vi "getColumn.vi"(0 "reference in":refnum<class "python.lvclass">, 1 "filePath":string, 2 "sheetName":string, 3 "column":string, 4 "row":string, 5 "error in (no error)":errorcluster) -> (14 "reference out":refnum<class "python.lvclass">, 16 "data":string[](array[string]), 19 "error out":errorcluster)   [LabVIEW 2015, in "python.lvclass"]
uses:
  python.lvclass
  <vilib>/Utility/error.llb/DialogType.ctl
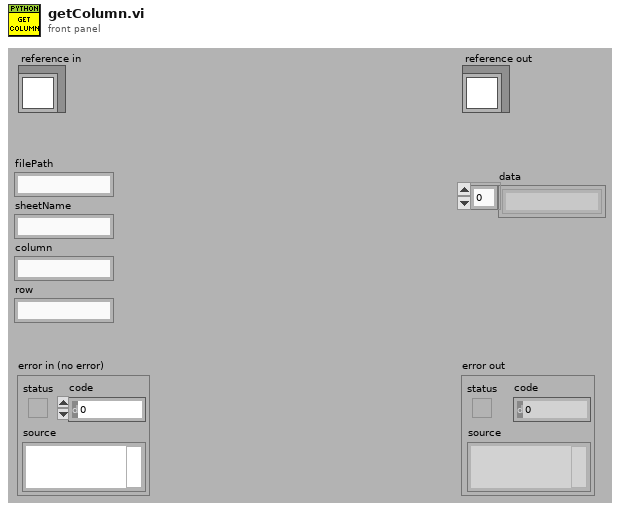
[diagram p1: front panel]
types:
  T1 = typedef "python.lvclass/ObjectAttributesRef.ctl" = refnum<data-value>
  T2 = typedef "python.lvclass/ObjectAttributes.ctl" = cluster{"MyAttribute":dbl, "workingDirectory":path}
  T3 = typedef "DialogType.ctl" = u16
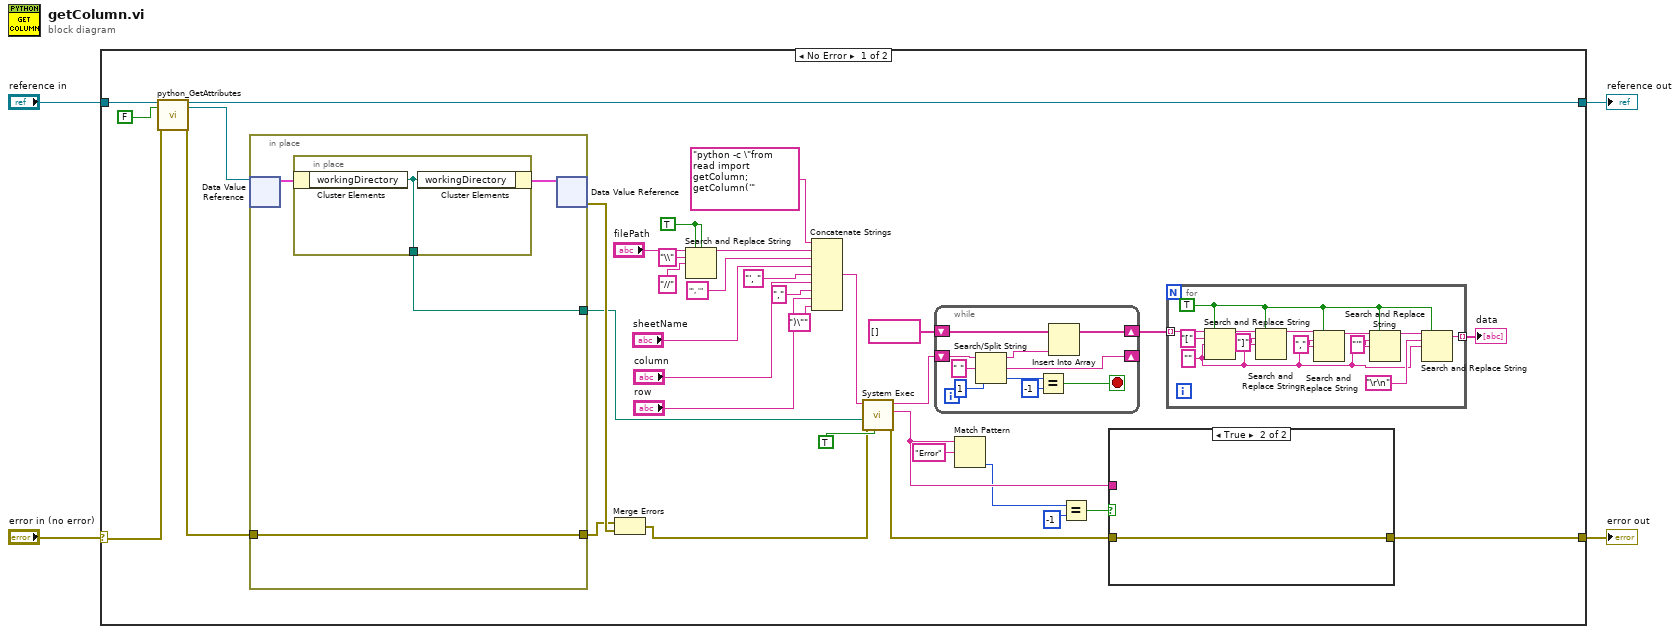
[diagram p0: block diagram]
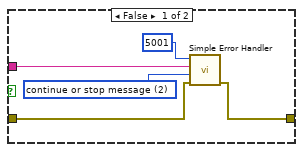
[diagram p2: hidden frame]
diagram:
  n1 = case shown="No Error" "error in (no error)" {
    selector: "error in (no error)" -> [w36 w76]
    tunnel: [w23 w76] -> w3
    tunnel: [w34 w75] -> w1
    tunnel: "reference in" -> [w38 w75]
    frame No Error {
      w18 = TRUE ("replace all? (F)")
      n2 = call "python_GetAttributes.vi"("reference in"=w38, "return data? (T)"=FALSE, "error in (no error)"=w36) -> ("reference out"=w34:refnum<class "python.lvclass">, "attributes ref"=w33:T1, "error out"=w35:errorcluster)  [unwired: 13 in, 1 out]
      n3 = in-place {
        in-place-border: w35 -> [w71]
        in-place-border: [w71] -> w39
        in-place-border: [w70] -> w31
        n4 = in-place-dvr #1(w33) -> (w72:T2)  [unwired: 1 out]
        n5 = in-place {
          in-place-border: [w74] -> w70
          n6 = in-place-cluster #2(w72) -> ("workingDirectory"=w74:path)
          n7 = in-place-cluster #2("workingDirectory"=w74) -> (w73:T2)
        }
        n8 = in-place-dvr #1(w73) -> (w40:errorcluster)  [unwired: 1 out]
      }
      n9 = Merge Errors(w39, w40) -> (w30:errorcluster)
      n10 = Search and Replace String(replace all?=w18, case sensitive?=w18, input string="filePath", search string="\\", replace string="//" ("search string")) -> (result string=w19:string)  [unwired: 3 in, 3 out]
      n11 = Concatenate Strings("python -c \"from read import getColumn; getColumn('" ("string"), w19, "', '" ("string"), "sheetName", "', " ("string"), "column", "," ("string"), "row", ")\"" ("string")) -> (w27:string)
      n12 = call <vilib>:"System Exec.vi"("run minimized? (F)"=TRUE, "error in (no error)"=w30, "working directory"=w31, "command line"=w27) -> ("error out"=w24:errorcluster, "standard error"=w17:string, "standard output"=w25:string)  [unwired: 2 in, 3 out]
      n13 = while {
        shift-right: [w68] -> w6
        shift-left: string[] [] -> [w69]
        shift-right: [w64] -> _
        shift-left: w25 -> [w67]
        stop <- w62 stop-if-true
        n14 = Search/Split String(string=w67, search string/char (-)=" ", offset (0)=1) -> (substring before match=w66:string, match + rest of string=w64:string, offset of match=w63:i32)
        n15 = Equal?(x=w63, y=-1) -> (x = y?=w62:bool)
        n16 = Insert Into Array(array=w69, new element=w66) -> (w68:string[])  [unwired: 1 in]
      }
      n17 = Match Pattern(string=w17, regular expression="Error") -> (offset past match=w13:i32)  [unwired: 1 in, 3 out]
      n18 = Equal?(x=w13, y=-1 ("offset past match")) -> (x = y?=w14:bool)
      n19 = case shown="True" w14 {
        tunnel: w24 -> [w58 w59]
        tunnel: [w57 w59] -> w23
        tunnel: w17 -> [w55 _]
        frame False {
          w54 = T3 2 items=["no dialog", "OK message", "continue or stop message", "OK message + warnings", "continue/stop + warnings"] ("type of dialog (OK msg:1)")
          n20 = call <vilib>:"Simple Error Handler.vi"("error code (no error:0)"=5001, "error source (\" \")"=w55, "type of dialog (OK msg:1)"=w54, "error in (no error)"=w58) -> ("error out"=w57:errorcluster)  [unwired: 5 out]
        }
        frame True {
        }
      }
      n21 = for {
        tunnel: w6 -> [w53] mode=indexing
        tunnel: [w41] -> w5 mode=indexing
        w42 = TRUE ("replace all? (F)")
        w43 = "" ("replace string (\"\")")
        n22 = Search and Replace String(replace all?=w42, input string=w53, search string="[", replace string=w43) -> (result string=w51:string)  [unwired: 4 in, 3 out]
        n23 = Search and Replace String(replace all?=w42, input string=w51, search string="]", replace string=w43) -> (result string=w48:string)  [unwired: 4 in, 3 out]
        n24 = Search and Replace String(replace all?=w42, input string=w48, search string=",", replace string=w43) -> (result string=w46:string)  [unwired: 4 in, 3 out]
        n25 = Search and Replace String(replace all?=w42, input string=w46, search string="'", replace string=w43) -> (result string=w45:string)  [unwired: 4 in, 3 out]
        n26 = Search and Replace String(replace all?=w42, input string=w45, search string="\r\n", replace string=w43) -> (result string=w41:string)  [unwired: 4 in, 3 out]
      }
      "data" <- w5
    }
    frame Error {
    }
  }
  "error out" <- w3
  "reference out" <- w1
